vi "21 Symmetrical Components (x64-2018).vi"(0 "Amplitude":dynamicdata(waveform), 1 "Phase":dynamicdata(waveform)) -> (2 "V0":dbl format="%.3f", 3 "Theta2":dbl, 4 "V1":dbl format="%.3f", 5 "V2":dbl format="%.3f", 6 "Theta0":dbl, 7 "Theta1":dbl)   [LabVIEW 2017]
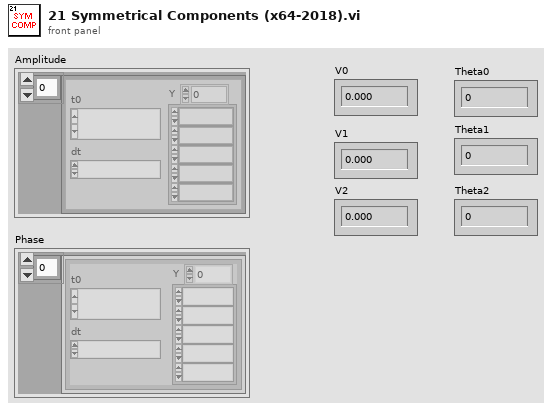
[diagram p1: front panel]
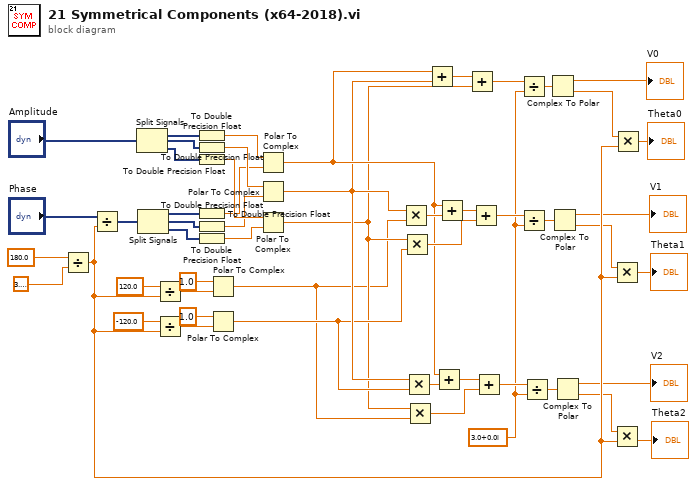
[diagram p0: block diagram]
diagram:
  w3 = cdb 3.0+0.0i ("y")
  n1 = Divide(x=180.0, y=3.141592653589793) -> (x/y=w23:dbl)
  n2 = Divide(x="Phase", y=w23) -> (x/y=w42:dynamicdata)
  n3 = Split Signals("Amplitude") -> (w52:dynamicdata, w50:dynamicdata, w48:dynamicdata)  [unwired: 3 in]
  n4 = Split Signals(w42) -> (w51:dynamicdata, w49:dynamicdata, w47:dynamicdata)  [unwired: 3 in]
  n5 = Divide(x=120.0, y=w23) -> (x/y=w28:dbl)
  n6 = Divide(x=-120.0, y=w23) -> (x/y=w25:dbl)
  n7 = To Double Precision Float(number=w52) -> (double precision float=w35:dbl)
  n8 = To Double Precision Float(number=w50) -> (double precision float=w34:dbl)
  n9 = To Double Precision Float(number=w48) -> (double precision float=w33:dbl)
  n10 = To Double Precision Float(number=w51) -> (double precision float=w32:dbl)
  n11 = To Double Precision Float(number=w49) -> (double precision float=w31:dbl)
  n12 = To Double Precision Float(number=w47) -> (double precision float=w30:dbl)
  n13 = Polar To Complex(1:w28, 2:1.0 ("r")) -> (0:w8:cdb)
  n14 = Polar To Complex(1:w25, 2:1.0 ("r")) -> (0:w10:cdb)
  n15 = Polar To Complex(1:w32, 2:w35) -> (0:w12:cdb)
  n16 = Polar To Complex(1:w31, 2:w34) -> (0:w11:cdb)
  n17 = Polar To Complex(1:w30, 2:w33) -> (0:w9:cdb)
  n18 = Multiply(x=w11, y=w8) -> (x*y=w19:cdb)
  n19 = Multiply(x=w9, y=w10) -> (x*y=w18:cdb)
  n20 = Multiply(x=w11, y=w10) -> (x*y=w14:cdb)
  n21 = Multiply(x=w9, y=w8) -> (x*y=w13:cdb)
  n22 = Add(x=w12, y=w11) -> (x+y=w46:cdb)
  n23 = Add(x=w12, y=w14) -> (x+y=w17:cdb)
  n24 = Add(x=w12, y=w19) -> (x+y=w22:cdb)
  n25 = Add(x=w46, y=w9) -> (x+y=w45:cdb)
  n26 = Add(x=w22, y=w18) -> (x+y=w21:cdb)
  n27 = Add(x=w17, y=w13) -> (x+y=w16:cdb)
  n28 = Divide(x=w45, y=w3) -> (x/y=w44:cdb)
  n29 = Divide(x=w21, y=w3) -> (x/y=w20:cdb)
  n30 = Divide(x=w16, y=w3) -> (x/y=w15:cdb)
  n31 = Complex To Polar(r * e^(i*theta)=w44) -> (r=→"V0":dbl, theta=w36:dbl)
  n32 = Complex To Polar(r * e^(i*theta)=w20) -> (r=→"V1":dbl, theta=w5:dbl)
  n33 = Complex To Polar(r * e^(i*theta)=w15) -> (r=→"V2":dbl, theta=w6:dbl)
  n34 = Multiply(x=w5, y=w23) -> (x*y=→"Theta1":dbl)
  n35 = Multiply(x=w6, y=w23) -> (x*y=→"Theta2":dbl)
  n36 = Multiply(x=w36, y=w23) -> (x*y=→"Theta0":dbl)
